vi "Commit Write.vi"(7 "Semaphore":T1, 8 "error in (no error)":errorcluster, 9 "Leave File Open?":bool, 11 "Configuration File In":refnum<class "Configuration File.lvclass">) -> (0 "error out":errorcluster, 3 "Configuration File Out":refnum<class "Configuration File.lvclass">)   [LabVIEW 2020, in "Configuration File.lvclass"]
uses:
  Configuration File.lvclass
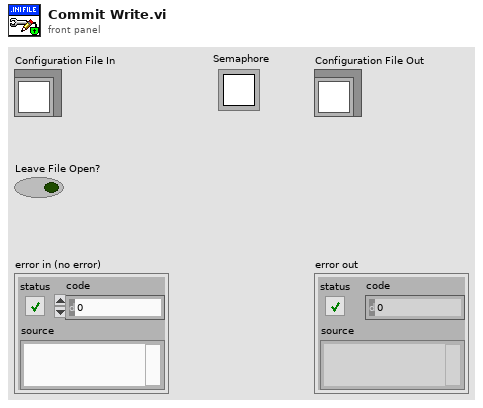
[diagram p1: front panel]
types:
  T1 = typedef "Semaphore RefNum" = refnum<k1>
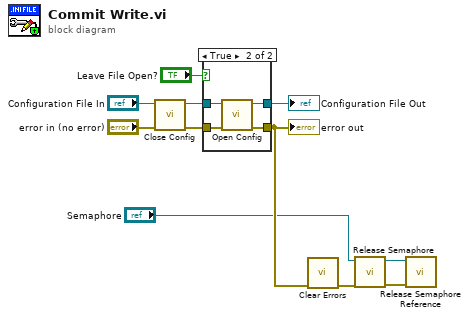
[diagram p0: block diagram]
diagram:
  n1 = call-dynamic "Close Config.vi"("error in (no error)"="error in (no error)", "Configuration File File In"="Configuration File In") -> ("error out"=w9:errorcluster, "Configuration File File Out"=w10:refnum<class "Configuration File.lvclass">)  [unwired: 8 in]
  n2 = case shown="True" "Leave File Open?" {
    tunnel: w9 -> [w13 w15]
    tunnel: [w13 w14] -> w2
    tunnel: w10 -> [w12 w17]
    tunnel: [w12 w16] -> w11
    frame False {
    }
    frame True {
      n3 = call-dynamic "Open Config.vi"("error in (no error)"=w15, "Configuration File File In"=w17) -> ("error out"=w14:errorcluster, "Configuration File File Out"=w16:refnum<class "Configuration File.lvclass">)  [unwired: 8 in]
    }
  }
  "Configuration File Out" <- w11
  "error out" <- w2
  n4 = call <vilib>:"Clear Errors.vi"("error in (no error)"=w2) -> ("error out"=w3:errorcluster)  [unwired: 5 in, 1 out]
  n5 = call <vilib>:"Release Semaphore.vi"("error in (no error)"=w3, "semaphore"="Semaphore") -> ("error out"=w4:errorcluster, "semaphore out"=w5:T1)  [unwired: 4 in]
  n6 = call <vilib>:"Release Semaphore Reference.vi"("error in (no error)"=w4, "semaphore"=w5) -> ()  [unwired: 8 in, 2 out]
